vi "Client DIO.vi"() -> ()   [LabVIEW 2015]
uses:
  <vilib>/MakerHub/LINX/Public/Peripherals/Digital/Digital Write 1 Chan.vi
  <vilib>/MakerHub/LINX/Public/Peripherals/Digital/Digital Read 1 Chan.vi
  <vilib>/MakerHub/LINX/LMH-LINX.lvlib
panel:
  in  "Connect":bool
  in  "About":bool
  in  "Stop":bool
  out "IO5":bool
  out "IO4":bool
  in  "IO3":bool
  in  "IO2":bool
  in  "VISA resource name":refnum<visa-resource-name>
  # "LabVIEW MakerHub"
  # "Proteus Test - Digital I/Os"
  # "COM Port"
  # "Output"
  # "Input"
  # "Quit"
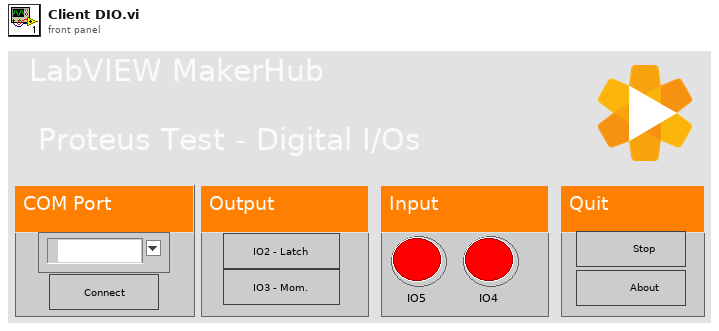
[diagram p1: front panel]
types:
  T1 = typedef "LMH-LINX.lvlib/LINX Ref.ctl" = cluster{"Platform":T2, "Interface":T3, "LINX Device Config":T4}
  T2 = typedef "LMH-LINX.lvlib/Platform.ctl" = enum16{"LINX", "myRIO"}
  T3 = typedef "LMH-LINX.lvlib/Interface.ctl" = enum16{"Serial", "TCP"}
  T4 = typedef "LMH-LINX.lvlib/Device.lvlib/LINX Device Config.ctl" = cluster{"Interface":T3, "COM Port":refnum<visa-resource-name>, "TCP Configuration":T5, "Device Family":u8, "Device ID":u8, "Device Name":string, "TCP Ref":refnum<k5>, "Channels":T6}
  T5 = typedef "LMH-LINX.lvlib/Device.lvlib/TCP Config.ctl" = cluster{"IP Address":string, "Port":u16}
  T6 = typedef "LMH-LINX.lvlib/Channels.ctl" = cluster{"DI":u8[], "DO":u8[], "AI":u8[], "AO":u8[], "PWM":u8[], "QE":u8[], "UART":u8[], "I2C 2":u8[], "SPI":u8[], "CAN":u8[], "Servo":u8[], "AI Ref (V)":dbl, "AO Ref (V)":dbl, "AO Resolution (Bits)":u8}
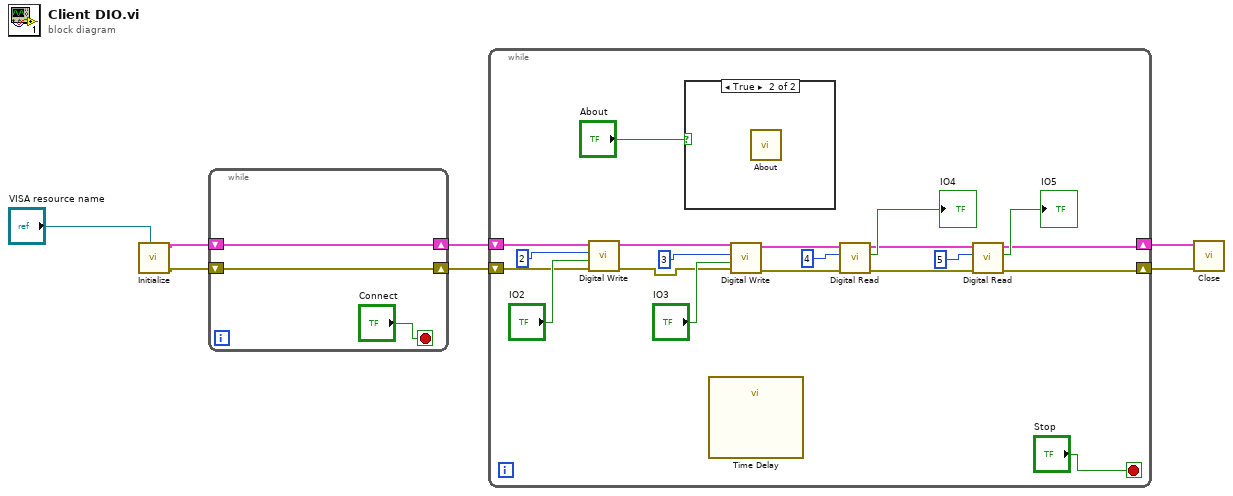
[diagram p0: block diagram]
diagram:
  n1 = call <vilib>:"Initialize.vi"("Serial Port"="VISA resource name") -> ("Error Out"=w1:errorcluster, "LINX Ref"=w2:T1)  [unwired: 8 in, 1 out]
  n2 = while {
    shift-right: [w9] -> w7
    shift-left: w2 -> [w9]
    shift-right: [w8] -> w6
    shift-left: w1 -> [w8]
    stop <- "Connect" stop-if-true
  }
  n3 = while {
    shift-right: [w14] -> w5
    shift-left: w7 -> [w30]
    shift-right: [w13] -> w4
    shift-left: w6 -> [w25]
    stop <- "Stop" stop-if-true
    n4 = call-poly <vilib>:"Digital Write.vi"("Error In"=w25, "Output Value"="IO2", "DO Channel"=u8 2, "LINX Resource"=w30) -> ("Error Out"=w24:errorcluster, "LINX Resource"=w23:T1)  [unwired: 6 in]
    n5 = case shown="True" "About" {
      frame False {
      }
      frame True {
        n6 = call "About.vi"() -> ()  [unwired: 1 in]
      }
    }
    n7 = call "Time Delay"() -> ()  [unwired: 11 in, 1 out]
    n8 = call-poly <vilib>:"Digital Write.vi"("Error In"=w24, "Output Value"="IO3", "DO Channel"=u8 3, "LINX Resource"=w23) -> ("Error Out"=w20:errorcluster, "LINX Resource"=w22:T1)  [unwired: 6 in]
    n9 = call-poly <vilib>:"Digital Read.vi"("Error In"=w20, "DI Channel"=u8 4, "LINX Resource"=w22) -> ("Error Out"=w17:errorcluster, "DI Value"=→"IO4":bool, "LINX Resource"=w18:T1)  [unwired: 6 in]
    n10 = call-poly <vilib>:"Digital Read.vi"("Error In"=w17, "DI Channel"=u8 5, "LINX Resource"=w18) -> ("Error Out"=w13:errorcluster, "DI Value"=→"IO5":bool, "LINX Resource"=w14:T1)  [unwired: 6 in]
  }
  n11 = call <vilib>:"Close.vi"("Error In"=w4, "LINX Resource"=w5) -> ()  [unwired: 8 in, 2 out]
